vi "Edit Sample.vi"(6 "Labels":map{string, string}(c390), 8 "error in (no error)":errorcluster, 9 "Action":T1=enum."Increment", 10 "Step":dbl, 11 "Metric in":refnum<class "Metric.lvclass">) -> (0 "error out":errorcluster, 2 "New Sample?":bool, 3 "Metric out":refnum<class "Metric.lvclass">)   [LabVIEW 2020, in "Metrics.lvlib" / "Metric.lvclass"]
doc: "Inserts or updates a sample corresponding to the labels passed as arguments. The sample value may be set or incremented"
uses:
  Metric.lvclass
  sample/Edit Action.ctl
  Metric.lvclass/Metric.ctl
  <vilib>/Utility/miscctls.llb/LVMapReplaceAction.ctl
  sample/Sample.lvclass
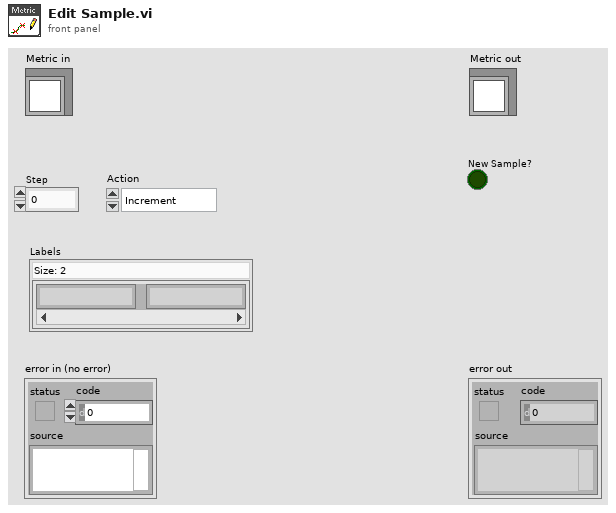
[diagram p1: front panel]
types:
  T1 = typedef "Metrics.lvlib/Sample.lvclass/Edit Action.ctl" = enum16{"Set", "Increment"}
  T2 = typedef "LVMapReplaceAction.ctl" = enum32{"Modify Entry only if found", "Add or Modify Entry", "Delete Entry"}
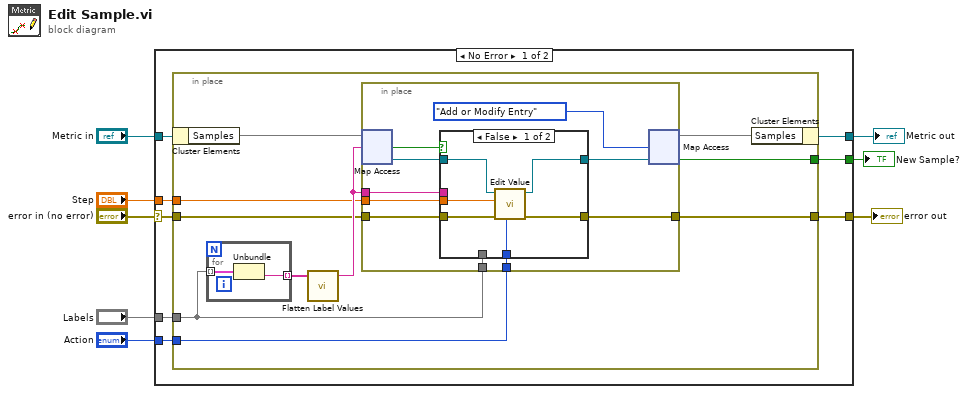
[diagram p0: block diagram]
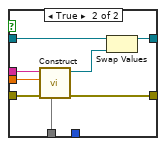
[diagram p2: hidden frame]
diagram:
  n1 = case shown="No Error" "error in (no error)" {
    selector: "error in (no error)" -> [w13 w54]
    tunnel: [w9 w54] -> w7
    tunnel: [w15 w53] -> w5
    tunnel: "Metric in" -> [w16 w53]
    tunnel: "Step" -> [w14 _]
    tunnel: "Labels" -> [w12 _]
    tunnel: "Action" -> [w11 _]
    tunnel: [w10 _] -> w2
    frame No Error {
      n2 = in-place {
        in-place-border: w14 -> [w24]
        in-place-border: w13 -> [w23]
        in-place-border: w12 -> [w18]
        in-place-border: w11 -> [w22]
        in-place-border: [w20] -> w10
        in-place-border: [w19] -> w9
        n3 = in-place-cluster #1(w16) -> ("Samples"=w25:map{string, refnum<class "Sample.lvclass">})
        n4 = for {
          tunnel: w18 -> [w52] mode=indexing
          tunnel: [w51] -> w17 mode=indexing
          n5 = Unbundle(w52) -> (w51:string)  [unwired: 1 out]
        }
        n6 = call "Flatten Label Values.vi"("Label Values"=w17) -> ("Flattened labelvalues"=w26:string)  [unwired: 4 in]
        n7 = in-place {
          in-place-border: w26 -> [w33]
          in-place-border: w24 -> [w32]
          in-place-border: w23 -> [w30]
          in-place-border: [w29] -> w19
          in-place-border: w18 -> [w28]
          in-place-border: w22 -> [w27]
          n8 = in-place-map #2(w25, w26) -> (w31:refnum<class "Sample.lvclass">, w35:bool)  [unwired: 1 in]
          n9 = case shown="False" w35 {
            tunnel: [w40 w47] -> w34
            tunnel: w33 -> [_ w50]
            tunnel: w32 -> [w38 w49]
            tunnel: w31 -> [w42 w46]
            tunnel: w30 -> [w41 w45]
            tunnel: [w39 w44] -> w29
            tunnel: w28 -> [_ w43]
            tunnel: w27 -> [w37 _]
            frame False {
              n10 = call "Edit Value.vi"("Action"=w37, "error in (no error)"=w41, "New Val"=w38, "Sample in"=w42) -> ("error out"=w39:errorcluster, "Sample out"=w40:refnum<class "Sample.lvclass">)  [unwired: 6 in]
            }
            frame True {
              n11 = call "Construct.vi"("Labels"=w43, "error in (no error)"=w45, "Value"=w49, "Name"=w50) -> ("error out"=w44:errorcluster, "Sample out"=w48:refnum<class "Sample.lvclass">)  [unwired: 6 in]
              n12 = Swap Values(12:w46, 14:w48) -> (1:w47:refnum<class "Sample.lvclass">)  [unwired: 1 in, 1 out]
            }
          }
          n13 = in-place-map #2(w34, LVMapReplaceAction."Add or Modify Entry" ("action")) -> (w21:map{string, refnum<class "Sample.lvclass">}, w20:bool)  [unwired: 1 out]
        }
        n14 = in-place-cluster #1("Samples"=w21) -> (w15:refnum<class "Metric.lvclass">)
      }
    }
    frame Error {
    }
  }
  "error out" <- w7
  "Metric out" <- w5
  "New Sample?" <- w2
